vi "API - Hardware in the Loop - Run Single Shot.vi"(8 "error in":errorcluster, 9 "Analog In Data Size":T1, 10 "Number of Samples":i32=80000, 11 "Analog Out Data":i16[][](array[numeric])) -> (0 "error out":errorcluster)   [LabVIEW 2017, in "DTACQ - Network Enabled Device Driver.lvlib"]
doc: "Captures a waveform (for each channel), using hardware in the loop mode"
uses:
  DTACQ - Network Enabled Device Driver.lvlib
  Communications/Typedefs/Data Size--Enum.ctl
  Close HIL Mode.vi
  Read HIL Data and Write to Shared Variable.vi
  Fire HIL Shot.vi
  Upload Analog Out Waveform.vi
  Initialise HIL Mode.vi
  Communications/Communications Library.lvlib
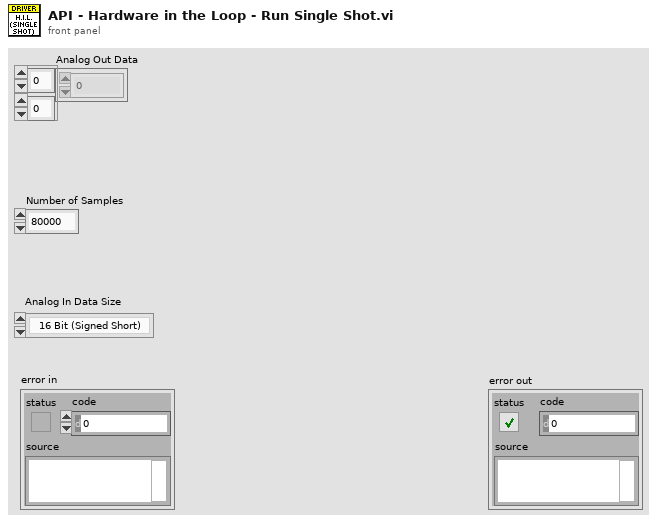
[diagram p1: front panel]
types:
  T1 = typedef "Communications Library.lvlib/Data Size--Enum.ctl" = enum16{"16 Bit (Signed Short)", "32 Bit (Signed Long)"}
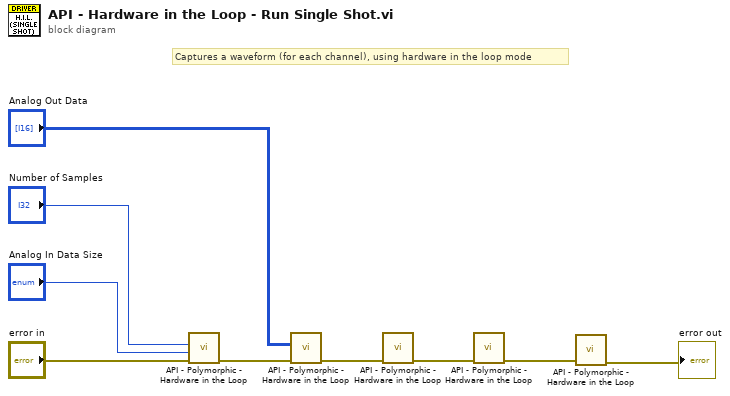
[diagram p0: block diagram]
diagram:
  # "Captures a waveform (for each channel), using hardware in the loop mode"
  n1 = call-poly "API - Polymorphic - Hardware in the Loop.vi"("error in"="error in", "Analog In Data Size"="Analog In Data Size", "Samples to Read"="Number of Samples") -> ("error out"=w6:errorcluster)  [unwired: 7 in, 1 out]
  n2 = call-poly "API - Polymorphic - Hardware in the Loop.vi"("error in"=w6, "Multichannel Waveform"="Analog Out Data") -> ("error out"=w4:errorcluster)  [unwired: 9 in]
  n3 = call-poly "API - Polymorphic - Hardware in the Loop.vi"("error in"=w4) -> ("error out"=w3:errorcluster)  [unwired: 9 in, 1 out]
  n4 = call-poly "API - Polymorphic - Hardware in the Loop.vi"("error in"=w3) -> ("error out"=w2:errorcluster)  [unwired: 10 in]
  n5 = call-poly "API - Polymorphic - Hardware in the Loop.vi"("error in"=w2) -> ("error out"=→"error out":errorcluster)  [unwired: 10 in]
